vi "ObtenerInformacionVariablesMotor.vi"(8 "error in (no error)":errorcluster) -> (0 "error out":errorcluster, 2 "Sucess?":bool, 3 "output cluster":T1)   [LabVIEW 2020, in "DataBaseSQLlite.lvlib"]
uses:
  DataBaseSQLlite.lvlib
  VariablesMotorTypeDef.ctl
  <vilib>/drjdpowell/SQLite Library/SQL Connection/Open (path).vi
  <vilib>/drjdpowell/SQLite Library/SQL Connection/Open (string).vi
  <vilib>/AdvancedString/Path To Command Line String.vi
  <vilib>/drjdpowell/SQLite Library/SQL Connection/Execute SQL (Single Integer).vi
  <vilib>/drjdpowell/SQLite Library/SQL Connection/Connection.lvclass
  <vilib>/drjdpowell/SQLite Library/SQLite.lvlib
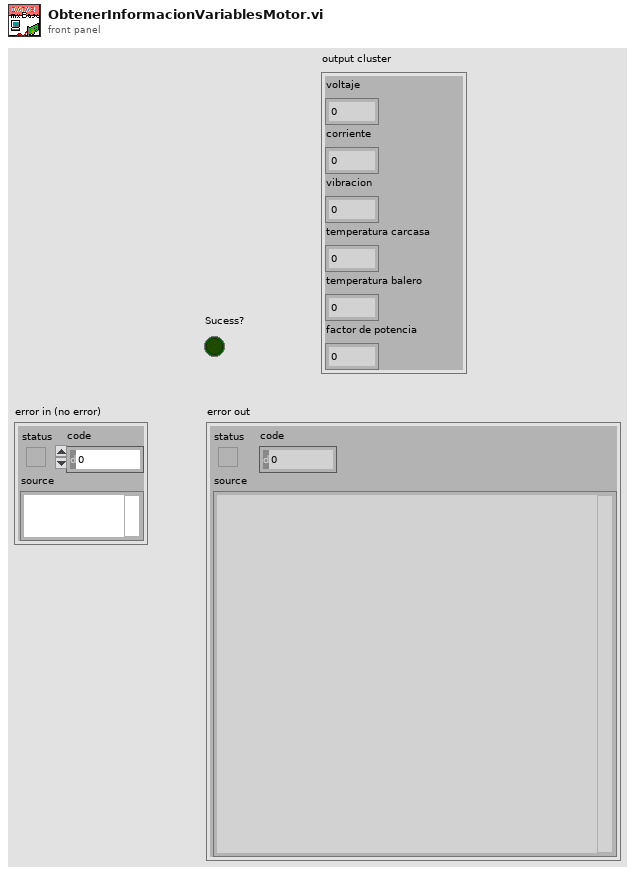
[diagram p1: front panel]
types:
  T1 = typedef "DataBaseSQLlite.lvlib/VariablesMotorTypeDef.ctl" = cluster{"voltaje":dbl, "corriente":dbl, "vibracion":dbl, "temperatura carcasa":dbl, "temperatura balero":dbl, "factor de potencia":dbl}
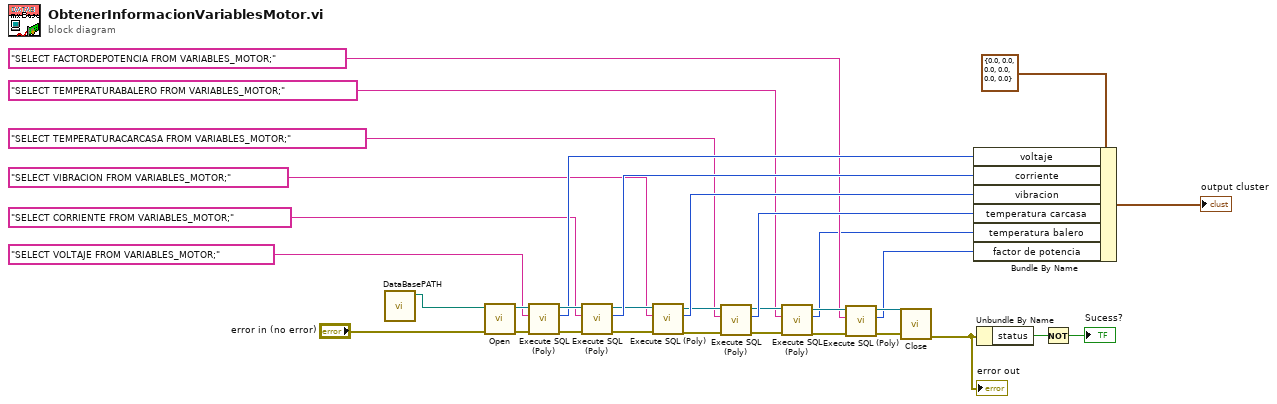
[diagram p0: block diagram]
diagram:
  n1 = call "DataBasePATH.vi"() -> ("DataBase path"=w33:path)  [unwired: 11 in]
  n2 = call-poly <vilib>:"Open.vi"("error in (no error)"="error in (no error)", "db file"=w33) -> ("error out"=w30:errorcluster, "SQLite Connection"=w31:refnum<class "Connection.lvclass">)  [unwired: 8 in]
  n3 = call-poly <vilib>:"Execute SQL (Poly).vi"("error in (no error)"=w30, "SQL"="SELECT VOLTAJE FROM VARIABLES_MOTOR;", "SQLite Connection in"=w31) -> ("error out"=w28:errorcluster, "Result"=w21:i64, "SQLite Connection"=w29:refnum<class "Connection.lvclass">)  [unwired: 6 in]
  n4 = call-poly <vilib>:"Execute SQL (Poly).vi"("error in (no error)"=w28, "SQL"="SELECT CORRIENTE FROM VARIABLES_MOTOR;", "SQLite Connection in"=w29) -> ("error out"=w17:errorcluster, "Result"=w19:i64, "SQLite Connection"=w18:refnum<class "Connection.lvclass">)  [unwired: 6 in]
  n5 = call-poly <vilib>:"Execute SQL (Poly).vi"("error in (no error)"=w17, "SQL"="SELECT VIBRACION FROM VARIABLES_MOTOR;", "SQLite Connection in"=w18) -> ("error out"=w13:errorcluster, "Result"=w15:i64, "SQLite Connection"=w14:refnum<class "Connection.lvclass">)  [unwired: 6 in]
  n6 = call-poly <vilib>:"Execute SQL (Poly).vi"("error in (no error)"=w13, "SQL"="SELECT TEMPERATURACARCASA FROM VARIABLES_MOTOR;", "SQLite Connection in"=w14) -> ("error out"=w11:errorcluster, "Result"=w10:i64, "SQLite Connection"=w9:refnum<class "Connection.lvclass">)  [unwired: 6 in]
  n7 = call-poly <vilib>:"Execute SQL (Poly).vi"("error in (no error)"=w11, "SQL"="SELECT TEMPERATURABALERO FROM VARIABLES_MOTOR;", "SQLite Connection in"=w9) -> ("error out"=w4:errorcluster, "Result"=w2:i64, "SQLite Connection"=w5:refnum<class "Connection.lvclass">)  [unwired: 6 in]
  n8 = call-poly <vilib>:"Execute SQL (Poly).vi"("error in (no error)"=w4, "SQL"="SELECT FACTORDEPOTENCIA FROM VARIABLES_MOTOR;", "SQLite Connection in"=w5) -> ("error out"=w7:errorcluster, "Result"=w1:i64, "SQLite Connection"=w6:refnum<class "Connection.lvclass">)  [unwired: 6 in]
  n9 = call-dynamic "Close.vi"("error in (no error)"=w7, "SQLite Connection in"=w6) -> ("error out"=w27:errorcluster)  [unwired: 9 in]
  "error out" <- w27
  n10 = Bundle By Name(cluster=T1 {"voltaje"=0.0, "corriente"=0.0, "vibracion"=0.0, "temperatura carcasa"=0.0, "temperatura balero"=0.0, "factor de potencia"=0.0} ("variables motor"), "voltaje"=w21, "corriente"=w19, "vibracion"=w15, "temperatura carcasa"=w10, "temperatura balero"=w2, "factor de potencia"=w1) -> (→"output cluster":T1)
  n11 = Unbundle By Name(w27) -> ("status"=w26:bool)
  n12 = Not(x=w26) -> (.not. x?=→"Sucess?":bool)
